vi "List Glyphs.vi"(8 "error in (no error)":errorcluster, 11 "Glyph Source in":refnum<class "Glyph Source.lvclass">) -> (0 "error out":errorcluster, 2 "Glyphs":string[](array[string]), 3 "Glyph Source out":refnum<class "Glyph Source.lvclass">)   [LabVIEW 2023, in "Font Glyph Drawer Interface.lvlib" / "Glyph Source.lvclass"]
uses:
  Glyph Source.lvclass
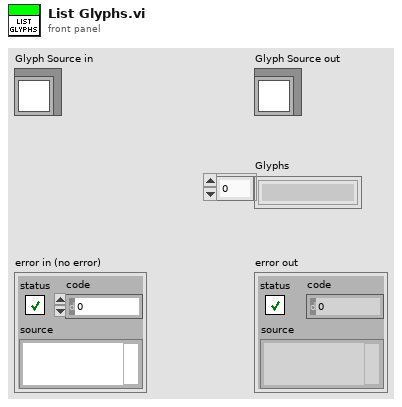
[diagram p1: front panel]
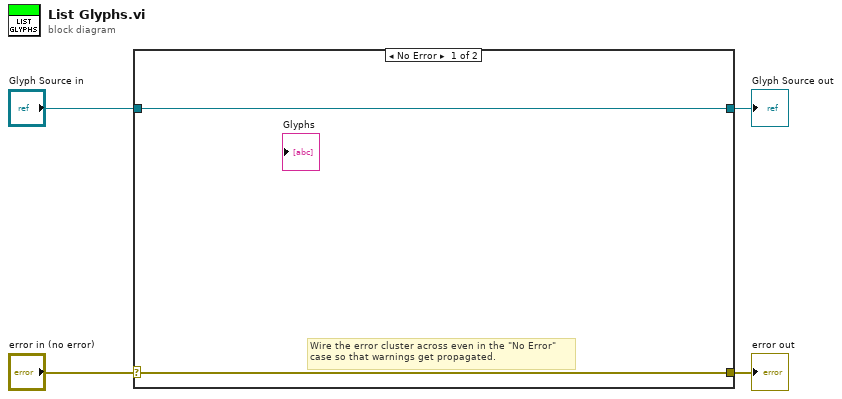
[diagram p0: block diagram]
diagram:
  n1 = case shown="No Error" "error in (no error)" {
    selector: "error in (no error)" -> [w5 w8]
    tunnel: [w5 w8] -> w3
    tunnel: [w6 w7] -> w1
    tunnel: "Glyph Source in" -> [w6 w7]
    frame No Error {
      # "Wire the error cluster across even in the \"No Error\"\ncase so that warnings get propagated."
    }
    frame Error {
    }
  }
  "error out" <- w3
  "Glyph Source out" <- w1
